vi "inout counter (SubVI).vi"(0 "Refnum in":refnum<k21>, 1 "Boolean 8":bool, 2 "Boolean 7":bool, 3 "Boolean 6":bool, 4 "Boolean 5":bool, 5 "Numeric 4":i32, 6 "Numeric 3":i32, 8 "stop in":bool, 10 "task in":refnum<k21>) -> (14 "task out":refnum<k21>, 16 "Boolean":bool, 17 "OUT COUNT":dbl, 18 "stop out":bool, 19 "IN ROOM":dbl, 20 "Refnum out":refnum<k21>, 21 "Boolean 2":bool, 22 "Boolean 4":bool, 23 "Boolean 3":bool, 24 "Numeric 2":i32, 25 "Numeric":i32, 26 "IN COUNT":dbl)   [LabVIEW 2022 SP3]
uses:
  <vilib>/DAQmx/read.llb/DAQmx Read (Digital Bool 1Line 1Point).vi
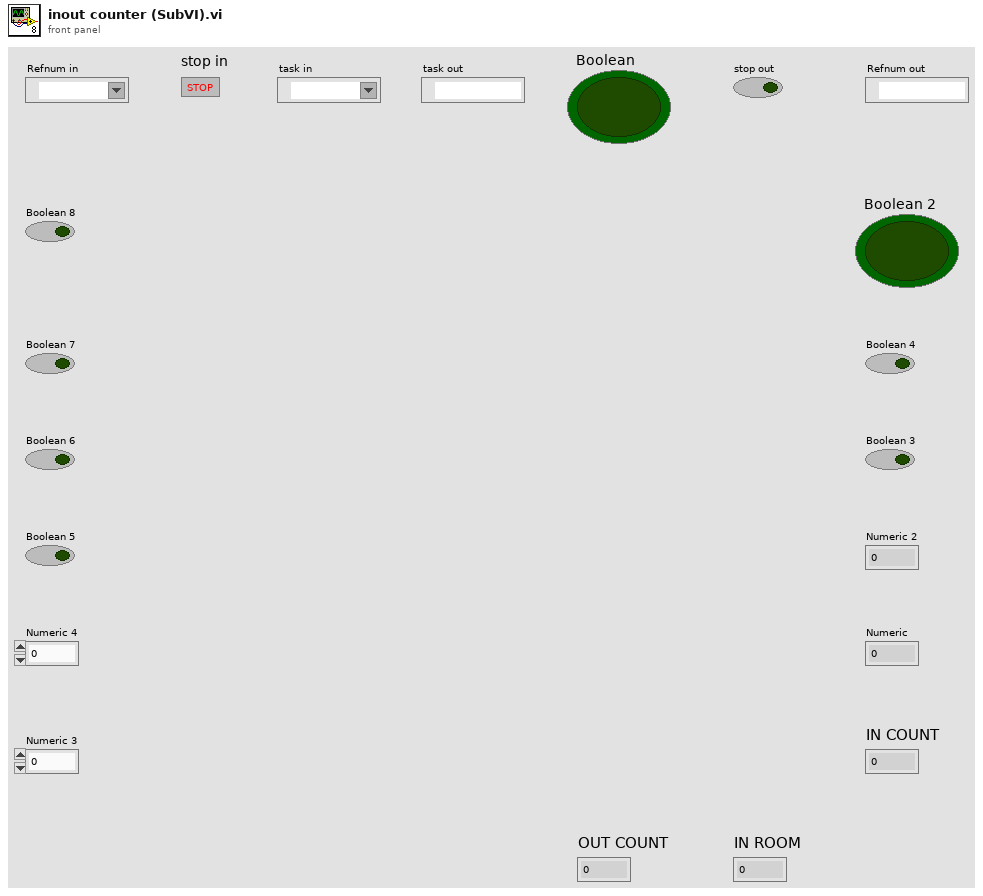
[diagram p1: front panel]
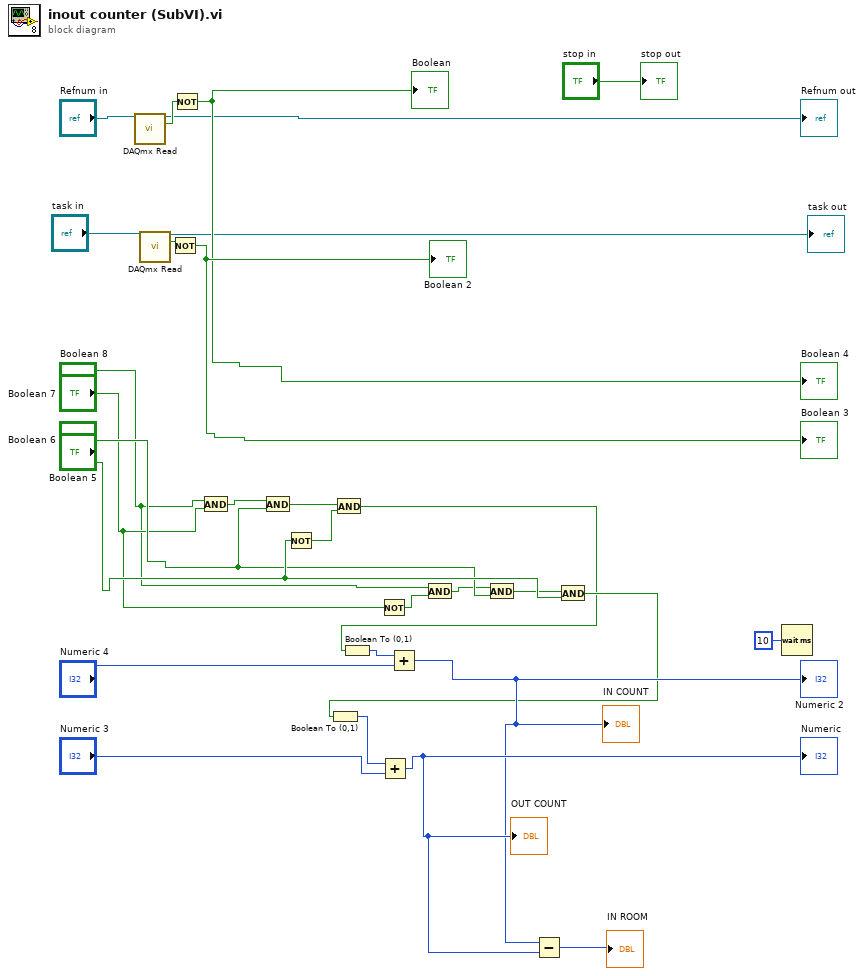
[diagram p0: block diagram]
diagram:
  n1 = call-poly <vilib>:"DAQmx Read.vi"("task/channels in"="Refnum in") -> ("task out"=→"Refnum out":refnum<k21>, "data"=w7:bool)  [unwired: 12 in, 1 out]
  n2 = call-poly <vilib>:"DAQmx Read.vi"("task/channels in"="task in") -> ("task out"=→"task out":refnum<k21>, "data"=w8:bool)  [unwired: 12 in, 1 out]
  n3 = Not(x=w8) -> (.not. x?=→"Boolean 2" →"Boolean 3":bool)
  n4 = Not(x=w7) -> (.not. x?=→"Boolean" →"Boolean 4":bool)
  n5 = And(x="Boolean 8", y="Boolean 7") -> (x .and. y?=w9:bool)
  n6 = And(x=w9, y="Boolean 6") -> (x .and. y?=w10:bool)
  n7 = Not(x="Boolean 5") -> (.not. x?=w11:bool)
  n8 = And(x=w10, y=w11) -> (x .and. y?=w23:bool)
  n9 = Boolean To (0,1)(Boolean=w23) -> (0, 1=w19:i16)
  n10 = Not(x="Boolean 7") -> (.not. x?=w15:bool)
  n11 = Add(x=w19, y="Numeric 4") -> (x+y=w27:i32)
  "IN COUNT" <- w27
  "Numeric 2" <- w27
  n12 = And(x="Boolean 8", y=w15) -> (x .and. y?=w12:bool)
  n13 = And(x=w12, y="Boolean 6") -> (x .and. y?=w13:bool)
  n14 = And(x=w13, y="Boolean 5") -> (x .and. y?=w25:bool)
  n15 = Boolean To (0,1)(Boolean=w25) -> (0, 1=w24:i16)
  n16 = Add(x=w24, y="Numeric 3") -> (x+y=w28:i32)
  "OUT COUNT" <- w28
  "Numeric" <- w28
  n17 = Subtract(x=w27, y=w28) -> (x-y=→"IN ROOM":i32)
  n18 = Wait (ms)(milliseconds to wait=u32 10) -> ()  [unwired: 1 out]
  "stop out" <- "stop in"
